vi "Sub02_PixmapBin.vi"(8 "error in (no error)":errorcluster, 9 "String":string, 10 "path in":path) -> (0 "error out":errorcluster, 5 "new picture":picture)   [LabVIEW 2019]
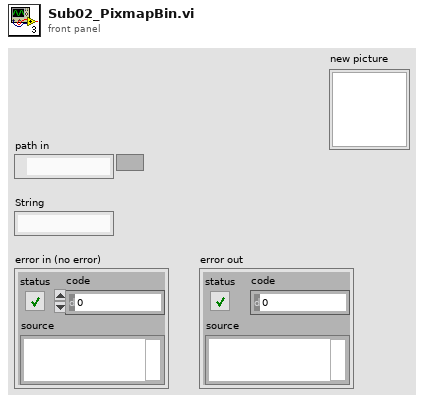
[diagram p1: front panel]
types:
  T1 = enum16{"big-endian, network order", "native, host order", "little-endian"}
  T2 = typedef "imagedata.ctl" = cluster{"image type":i32, "image depth":i32, "image":u8[], "mask":u8[], "colors":u32[], "Rectangle":cluster{"left":i16, "top":i16, "right":i16, "bottom":i16}}
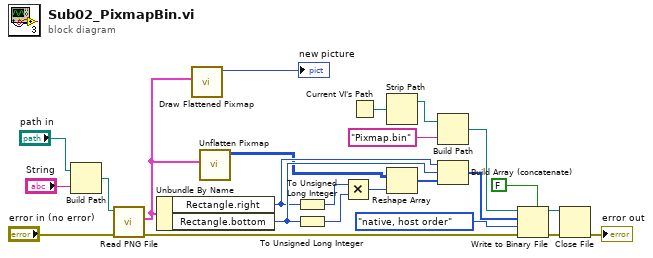
[diagram p0: block diagram]
diagram:
  n1 = Build Path(base path="path in", name or relative path="String") -> (appended path=w7:path)
  n2 = call <vilib>:"Read PNG File.vi"("error in (no error)"="error in (no error)", "path to PNG file"=w7) -> ("error out"=w9:errorcluster, "image data"=w4:T2)  [unwired: 7 in, 1 out]
  n3 = Unbundle By Name(w4) -> ("Rectangle.right"=w16:i16, "Rectangle.bottom"=w17:i16)
  n4 = call <vilib>:"Draw Flattened Pixmap.vi"("image data"=w4) -> ("new picture"=→"new picture":picture)  [unwired: 8 in]
  n5 = call <vilib>:"Unflatten Pixmap.vi"("image data"=w4) -> ("24-bit pixmap"=w10:u32[][])  [unwired: 4 in, 6 out]
  n6 = To Unsigned Long Integer(number=w16) -> (unsigned 32bit integer=w12:u32)
  n7 = To Unsigned Long Integer(number=w17) -> (unsigned 32bit integer=w13:u32)
  n8 = Multiply(x=w12, y=w13) -> (x*y=w14:u32)
  n9 = Current VI's Path() -> (path=w2:path)
  n10 = Strip Path(path=w2) -> (stripped path=w1:path)  [unwired: 1 out]
  n11 = Reshape Array(w10, w14) -> (w15:u32[])
  n12 = Build Path(base path=w1, name or relative path="Pixmap.bin") -> (appended path=w23:path)
  n13 = Build Array (concatenate)(w16, w17, w15) -> (w18:u32[])
  n14 = Write to Binary File(file (use dialog)=w23, data=w18, error in=w9, 5:FALSE ("prepend array or string size? (T)"), 9:T1."native, host order" ("byte order (0:big-endian, network order)")) -> (refnum out=w22:refnum<file>, error out=w21:errorcluster)  [unwired: 1 in, 1 out]
  n15 = Close File(refnum=w22, error in=w21) -> (error out=→"error out":errorcluster)  [unwired: 1 out]
